vi "ColorMap_main.vi"(7 "StressDist_types":T9, 8 "Error In":errorcluster, 9 "RefCM":refnum<vi>, 10 "Deformed":bool, 11 "main_FGV_data":T1={"pipe_properties"={"out_radius"=0.0, "in_radius"=0.0, "out_diameter"=0.0, "in_diameter"=0.0, "thickness"=0.0, "inertia"=0.0, "area"=0.0}, "DirPath"=path "L:/Documentos/00 SERVIÇOS/Tensão residual/Olapa 10-2017/Dados/Primeira Seção/Furos", "DirReport"=path "L:/Documentos/00 SERVIÇOS/Tensão residual/Olapa 10-2017/RelatóriosOlapa/Teste", "Points"=[], "ovalization_data"={"AngOval"=[0.0, 60.0, 120.0, 22.5, 45.0, 67.5, 90.0, 112.5, 135.0, 157.5, 180.0], "OvalDiam"=[324.25, 324.6, 324.55, 324.25, 324.55, 324.65, 324.6, 324.65, 324.55, 324.5, 324.4], "Plots"={"Ref"={"X"=[], "Y"=[]}, "Elipse"={"X"=[], "Y"=[]}, "Points"={"X"=[], "Y"=[]}}, "Ampliation"=100.0, "Results"={"MD"=0.0, "mD"=0.0, "Dmed"=0.0, "Oval"=0.0, "ang"=0.0, "X0"=0.0, "Y0"=0.0}, "fit"=[]}, "StressDist_data"={"Long"={"Plot"=[], "Fit"=[], "ColorMap"=[], "Data"=[], "peirce_data"={"Plot"=[], "Index removidos"=[]}}, "Circ"={"Plot"=[], "Fit"=[], "ColorMap"=[], "Data"=[], "peirce_data"={"Plot"=[], "Index removidos"=[]}}, "Shear"={"Plot"=[], "Fit"=[], "ColorMap"=[], "Data"=[], "peirce_data"={"Plot"=[], "Index removidos"=[]}}, "Equivalent"={"Plot"=[], "Fit"=[], "ColorMap"=[], "Data"=[], "peirce_data"={"Plot"=[], "Index removidos"=[]}}}, "pressure_data"={"Pressure"=[], "StressCircOval"=[], "StressCirc"=[], "StressLong"=[], "Plot"=[], "Angle"=[]}, "Reload"=FALSE}) -> (0 "Error Out":errorcluster, 3 "main_FGV_data-out":T1={"pipe_properties"={"out_radius"=0.0, "in_radius"=0.0, "out_diameter"=0.0, "in_diameter"=0.0, "thickness"=0.0, "inertia"=0.0, "area"=0.0}, "DirPath"=path "L:/Documentos/00 SERVIÇOS/Tensão residual/Olapa 10-2017/Dados/Primeira Seção/Furos", "DirReport"=path "L:/Documentos/00 SERVIÇOS/Tensão residual/Olapa 10-2017/RelatóriosOlapa/Teste", "Points"=[], "ovalization_data"={"AngOval"=[0.0, 60.0, 120.0, 22.5, 45.0, 67.5, 90.0, 112.5, 135.0, 157.5, 180.0], "OvalDiam"=[324.25, 324.6, 324.55, 324.25, 324.55, 324.65, 324.6, 324.65, 324.55, 324.5, 324.4], "Plots"={"Ref"={"X"=[], "Y"=[]}, "Elipse"={"X"=[], "Y"=[]}, "Points"={"X"=[], "Y"=[]}}, "Ampliation"=100.0, "Results"={"MD"=0.0, "mD"=0.0, "Dmed"=0.0, "Oval"=0.0, "ang"=0.0, "X0"=0.0, "Y0"=0.0}, "fit"=[]}, "StressDist_data"={"Long"={"Plot"=[], "Fit"=[], "ColorMap"=[], "Data"=[], "peirce_data"={"Plot"=[], "Index removidos"=[]}}, "Circ"={"Plot"=[], "Fit"=[], "ColorMap"=[], "Data"=[], "peirce_data"={"Plot"=[], "Index removidos"=[]}}, "Shear"={"Plot"=[], "Fit"=[], "ColorMap"=[], "Data"=[], "peirce_data"={"Plot"=[], "Index removidos"=[]}}, "Equivalent"={"Plot"=[], "Fit"=[], "ColorMap"=[], "Data"=[], "peirce_data"={"Plot"=[], "Index removidos"=[]}}}, "pressure_data"={"Pressure"=[], "StressCircOval"=[], "StressCirc"=[], "StressLong"=[], "Plot"=[], "Angle"=[]}, "Reload"=FALSE})   [LabVIEW 2016]
uses:
  StressDist_types.ctl
  MainFGV/main_FGV_data.ctl
  MainFGV/pipe_properties.ctl
  StressCalculations/point_data.ctl
  Ovalization/ovalization_data.ctl
  StressDist_data.ctl
  StressDist_single_data.ctl
  Peirce/peirce_data.ctl
  Pressure/pressure_data.ctl
  <vilib>/Analysis/1siggen.llb/Ramp Pattern by Samples.vi
  <vilib>/Analysis/geometry.llb/Point in Polygon.vi
  <vilib>/Analysis/geometry.llb/Point in Polygon (Scalar).vi
  <vilib>/Analysis/NI_AALBase.lvlib
panel:
  in  "Config":bool
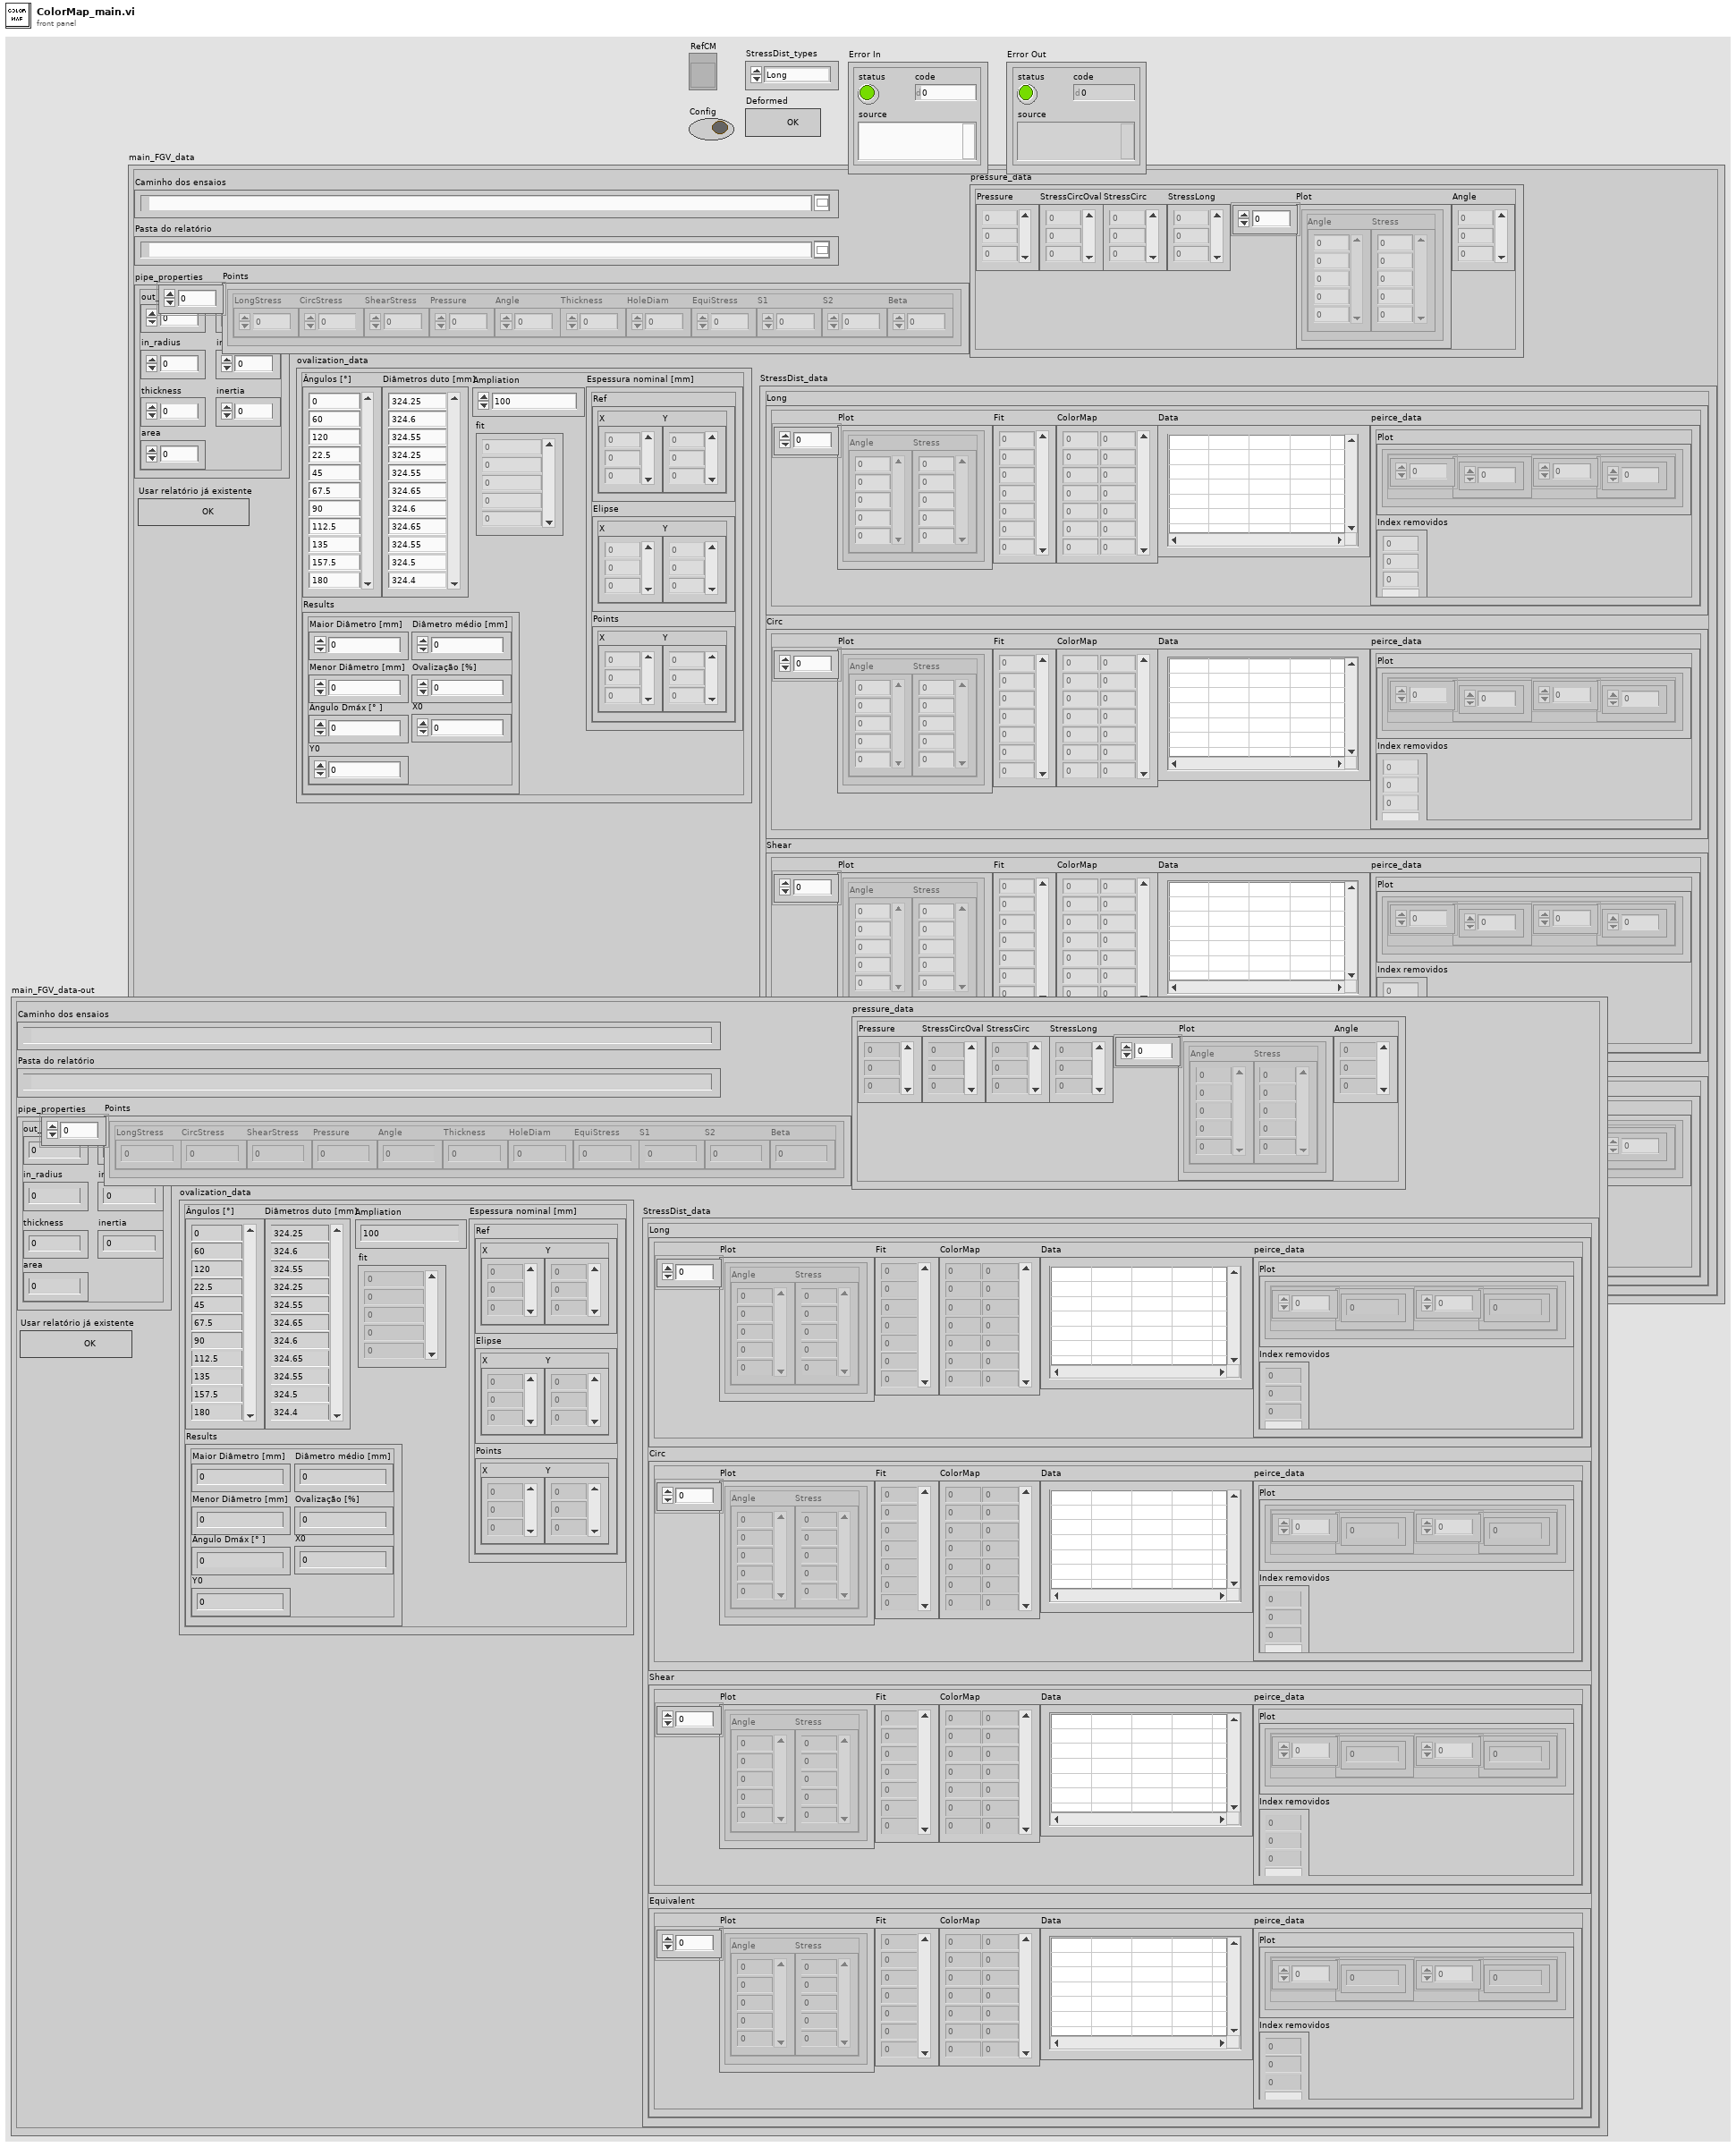
[diagram p1: front panel]
types:
  T1 = typedef "main_FGV_data.ctl" = cluster{"pipe_properties":T2, "DirPath":path, "DirReport":path, "Points":T3[], "ovalization_data":T4, "StressDist_data":T5, "pressure_data":T8, "Reload":bool}
  T2 = typedef "pipe_properties.ctl" = cluster{"out_radius":dbl, "in_radius":dbl, "out_diameter":dbl, "in_diameter":dbl, "thickness":dbl, "inertia":dbl, "area":dbl}
  T3 = typedef "point_data.ctl" = cluster{"LongStress":dbl, "CircStress":dbl, "ShearStress":dbl, "Pressure":dbl, "Angle":dbl, "Thickness":dbl, "HoleDiam":dbl, "EquiStress":dbl, "S1":dbl, "S2":dbl, "Beta":dbl}
  T4 = typedef "ovalization_data.ctl" = cluster{"AngOval":dbl[], "OvalDiam":dbl[], "Plots":cluster{"Ref":cluster{"X":dbl[], "Y":dbl[]}, "Elipse":cluster{"X":dbl[], "Y":dbl[]}, "Points":cluster{"X":dbl[], "Y":dbl[]}}, "Ampliation":dbl, "Results":cluster{"MD":dbl, "mD":dbl, "Dmed":dbl, "Oval":dbl, "ang":dbl, "X0":dbl, "Y0":dbl}, "fit":dbl[]}
  T5 = typedef "StressDist_data.ctl" = cluster{"Long":T6, "Circ":T6, "Shear":T6, "Equivalent":T6}
  T6 = typedef "StressDist_single_data.ctl" = cluster{"Plot":cluster{"Angle":dbl[], "Stress":dbl[]}[], "Fit":dbl[], "ColorMap":dbl[][], "Data":string[][], "peirce_data":T7}
  T7 = typedef "peirce_data.ctl" = cluster{"Plot":cluster{"Array":dbl[], "Array":dbl[]}[], "Index removidos":i32[]}
  T8 = typedef "pressure_data.ctl" = cluster{"Pressure":dbl[], "StressCircOval":dbl[], "StressCirc":dbl[], "StressLong":dbl[], "Plot":cluster{"Angle":dbl[], "Stress":dbl[]}[], "Angle":dbl[]}
  T9 = typedef "StressDist_types.ctl" = enum16{"Long", "Circ", "Shear", "Equivalent"}
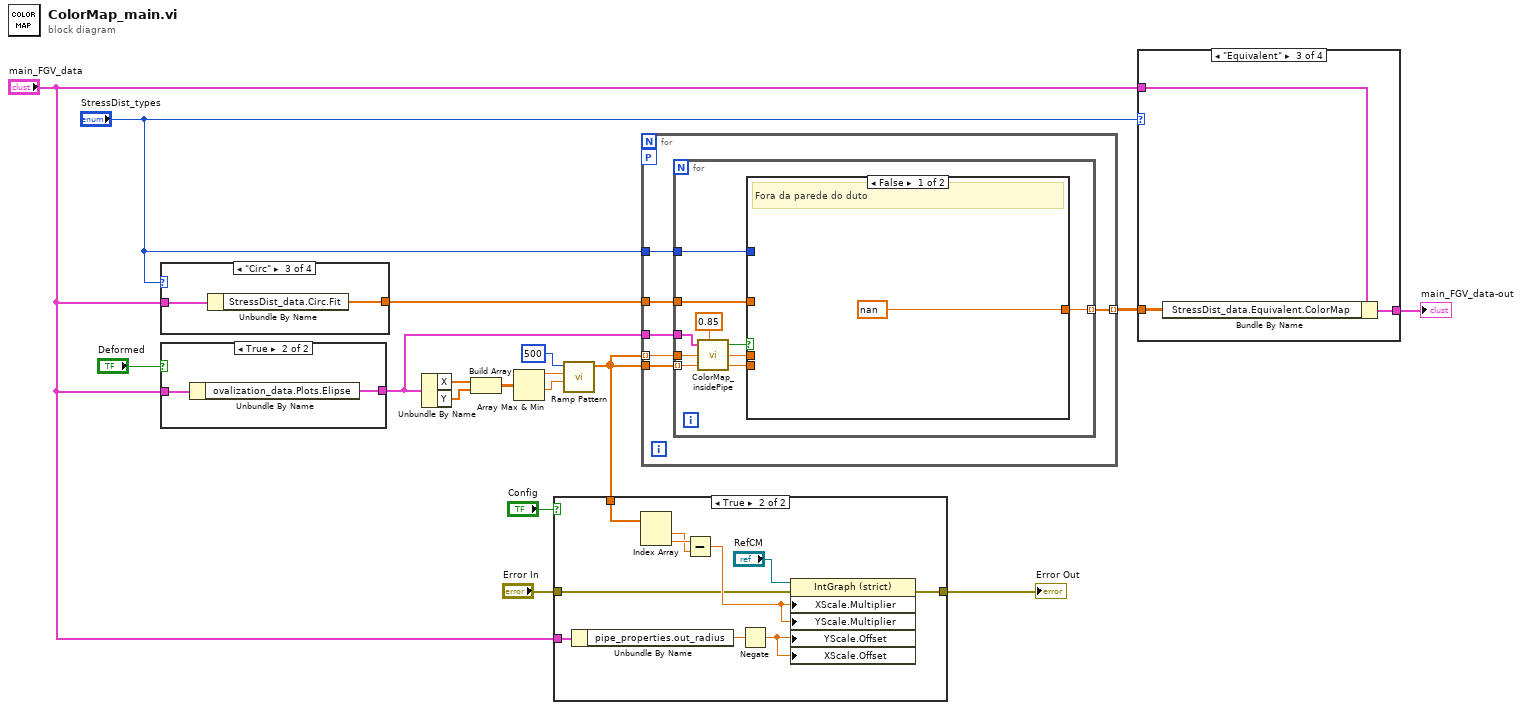
[diagram p0: block diagram]
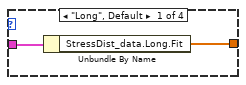
[diagram p3: hidden frame]
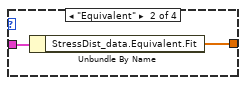
[diagram p4: hidden frame]
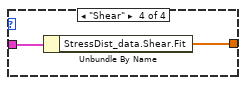
[diagram p5: hidden frame]
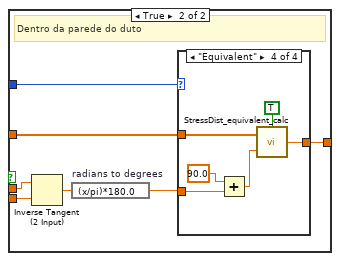
[diagram p6: hidden frame]
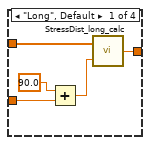
[diagram p7: hidden frame]
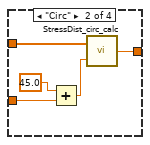
[diagram p8: hidden frame]
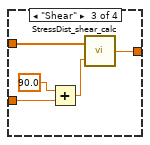
[diagram p9: hidden frame]
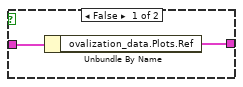
[diagram p10: hidden frame]
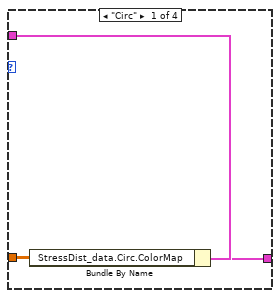
[diagram p11: hidden frame]
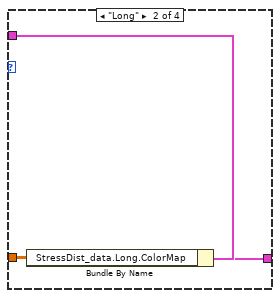
[diagram p12: hidden frame]
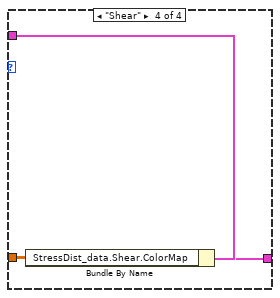
[diagram p13: hidden frame]
diagram:
  n1 = case shown="\"Circ\"" "StressDist_types" {
    tunnel: "main_FGV_data" -> [w19 w21 w23 w25]
    tunnel: [w18 w20 w22 w24] -> w10
    frame "Long", Default {
      n2 = Unbundle By Name(w19) -> ("StressDist_data.Long.Fit"=w18:dbl[])
    }
    frame "Equivalent" {
      n3 = Unbundle By Name(w21) -> ("StressDist_data.Equivalent.Fit"=w20:dbl[])
    }
    frame "Circ" {
      n4 = Unbundle By Name(w23) -> ("StressDist_data.Circ.Fit"=w22:dbl[])
    }
    frame "Shear" {
      n5 = Unbundle By Name(w25) -> ("StressDist_data.Shear.Fit"=w24:dbl[])
    }
  }
  n6 = case shown="True" "Deformed" {
    tunnel: "main_FGV_data" -> [w27 w29]
    tunnel: [w26 w28] -> w9
    frame False {
      n7 = Unbundle By Name(w27) -> ("ovalization_data.Plots.Ref"=w26:cluster{"X":dbl[], "Y":dbl[]})
    }
    frame True {
      n8 = Unbundle By Name(w29) -> ("ovalization_data.Plots.Elipse"=w28:cluster{"X":dbl[], "Y":dbl[]})
    }
  }
  n9 = Unbundle By Name(w9) -> ("X"=w16:dbl[], "Y"=w15:dbl[])
  n10 = Build Array(w16, w15) -> (w14:dbl[][])
  n11 = Array Max & Min(array=w14) -> (max value=w13:dbl, min value=w12:dbl)  [unwired: 2 out]
  n12 = call-poly <vilib>:"Ramp Pattern.vi"("start"=w12, "end"=w13, "samples"=500) -> ("Ramp Pattern"=w6:dbl[])  [unwired: 7 in, 1 out]
  n13 = case shown="True" "Config" {
    tunnel: w6 -> [_ w40]
    tunnel: "Error In" -> [w30 w35]
    tunnel: [w30 w34] -> w4
    tunnel: "main_FGV_data" -> [_ w33]
    frame False {
    }
    frame True {
      n14 = Unbundle By Name(w33) -> ("pipe_properties.out_radius"=w32:dbl)
      n15 = Index Array(array=w40) -> (element #1=w38:dbl, element #2=w39:dbl)  [unwired: 2 in]
      n16 = Subtract(x=w39, y=w38) -> (x-y=w37:dbl)
      n17 = Negate(x=w32) -> (-x=w31:dbl)
      n18 = property on="Property Node" class="IntGraph (strict)"(reference="RefCM", error in=w35, "XScale.Multiplier"=w37, "YScale.Multiplier"=w37, "YScale.Offset"=w31, "XScale.Offset"=w31) -> (error out=w34:errorcluster)  [unwired: 1 out]
    }
  }
  "Error Out" <- w4
  n19 = for {
    tunnel: w6 -> [w46] mode=indexing
    tunnel: w6 -> [w45]
    tunnel: "StressDist_types" -> [w44]
    tunnel: w10 -> [w43]
    tunnel: w9 -> [w42]
    tunnel: [w41] -> w1 mode=indexing
    workers-P: _ -> [_]
    n20 = for {
      tunnel: w46 -> [w47]
      tunnel: w45 -> [w48] mode=indexing
      tunnel: w44 -> [w56]
      tunnel: w43 -> [w55]
      tunnel: w42 -> [w52]
      tunnel: [w49] -> w41 mode=indexing
      n21 = call "ColorMap_insidePipe.vi"("Shape"=w52, "RedFactor"=0.85, "Yin"=w47, "Xin"=w48) -> ("Inside"=w50:bool, "Yout"=w54:dbl, "Xout"=w53:dbl)  [unwired: 1 in]
      n22 = case shown="False" w50 {
        tunnel: w56 -> [_ w64]
        tunnel: w55 -> [_ w63]
        tunnel: w54 -> [_ w62]
        tunnel: w53 -> [_ w61]
        tunnel: [nan ("Stress") w60] -> w49
        frame False {
          # "Fora da parede do duto"
        }
        frame True {
          # "Dentro da parede do duto"
          n23 = Inverse Tangent (2 Input)(1:w61, 2:w62) -> (0:w58:dbl)
          n24 = expression code="(x/pi)*180.0" "radians to degrees"(w58) -> (w59:dbl)
          n25 = case shown="\"Equivalent\"" w64 {
            tunnel: w63 -> [w69 w74 w79 w85]
            tunnel: w59 -> [w66 w72 w76 w82]
            tunnel: [w68 w73 w78 w84] -> w60
            frame "Long", Default {
              n26 = Add(x=90.0, y=w66) -> (x+y=w65:dbl)
              n27 = call "StressDist_long_calc.vi"("Angle"=w65, "Parameters"=w69) -> ("Stress"=w68:dbl)
            }
            frame "Circ" {
              n28 = Add(x=45.0, y=w72) -> (x+y=w71:dbl)
              n29 = call "StressDist_circ_calc.vi"("Angle"=w71, "Parameters"=w74) -> ("Stress"=w73:dbl)
            }
            frame "Shear" {
              n30 = Add(x=90.0, y=w76) -> (x+y=w75:dbl)
              n31 = call "StressDist_shear_calc.vi"("Angle"=w75, "Parameters"=w79) -> ("Stress"=w78:dbl)
            }
            frame "Equivalent" {
              n32 = Add(x=90.0, y=w82) -> (x+y=w81:dbl)
              n33 = call "StressDist_equivalent_calc.vi"("ColorMap?"=TRUE, "Angle"=w81, "Parameters"=w85) -> ("Stress"=w84:dbl)
            }
          }
        }
      }
    }
  }
  n34 = case shown="\"Equivalent\"" "StressDist_types" {
    tunnel: "main_FGV_data" -> [w88 w91 w94 w97]
    tunnel: w1 -> [w87 w90 w93 w96]
    tunnel: [w86 w89 w92 w95] -> w7
    frame "Circ" {
      n35 = Bundle By Name(cluster=w88, "StressDist_data.Circ.ColorMap"=w87) -> (w86:T1)
    }
    frame "Long" {
      n36 = Bundle By Name(cluster=w91, "StressDist_data.Long.ColorMap"=w90) -> (w89:T1)
    }
    frame "Equivalent" {
      n37 = Bundle By Name(cluster=w94, "StressDist_data.Equivalent.ColorMap"=w93) -> (w92:T1)
    }
    frame "Shear" {
      n38 = Bundle By Name(cluster=w97, "StressDist_data.Shear.ColorMap"=w96) -> (w95:T1)
    }
  }
  "main_FGV_data-out" <- w7
